vi "Periodic Tasks.vi"(8 "error in (no error)":errorcluster) -> ()   [LabVIEW 2012]
doc: "This VI runs in parallel to other tasks. It can contain as many user-defined periodic loops as you need. These can carry out PID or other sorts of timed response."
uses:
  <vilib>/Rock Robotics/WPI/Joystick/WPI_JoystickButtonState.ctl
  <vilib>/Rock Robotics/WPI/Solenoid/WPI_SolenoidValue.ctl
  <vilib>/Rock Robotics/SystemInterfaces/Utilities/FPGA_UtilitiesLED Source.ctl
  <vilib>/Rock Robotics/SystemInterfaces/Utilities/FPGA_UtilitiesLED State.ctl
  Robot Global Data.vi
  <vilib>/Rock Robotics/WPI/Solenoid/WPI_SolenoidSetEnum.vi
  <vilib>/Rock Robotics/WPI/Joystick/WPI_JoystickGetSetRefNum.vi
  <vilib>/Rock Robotics/WPI/RobotDrive/WPI_RobotDriveGetSetRefNum.vi
  <vilib>/Rock Robotics/WPI/RobotDrive/WPI_RobotDriveArcadeDrive_Standard(NoSaturation).vi
  <vilib>/Rock Robotics/WPI/Compressor/WPI_CompressorGetSetRefNum.vi
panel:
  out "Axes":T1
  out "Buttons":T2
  out "Voltage":dbl
  out "Emergency Stop":bool
  out "rear":bool
  out "front":bool
  out "Right Rear":bool
  out "Left Rear":bool
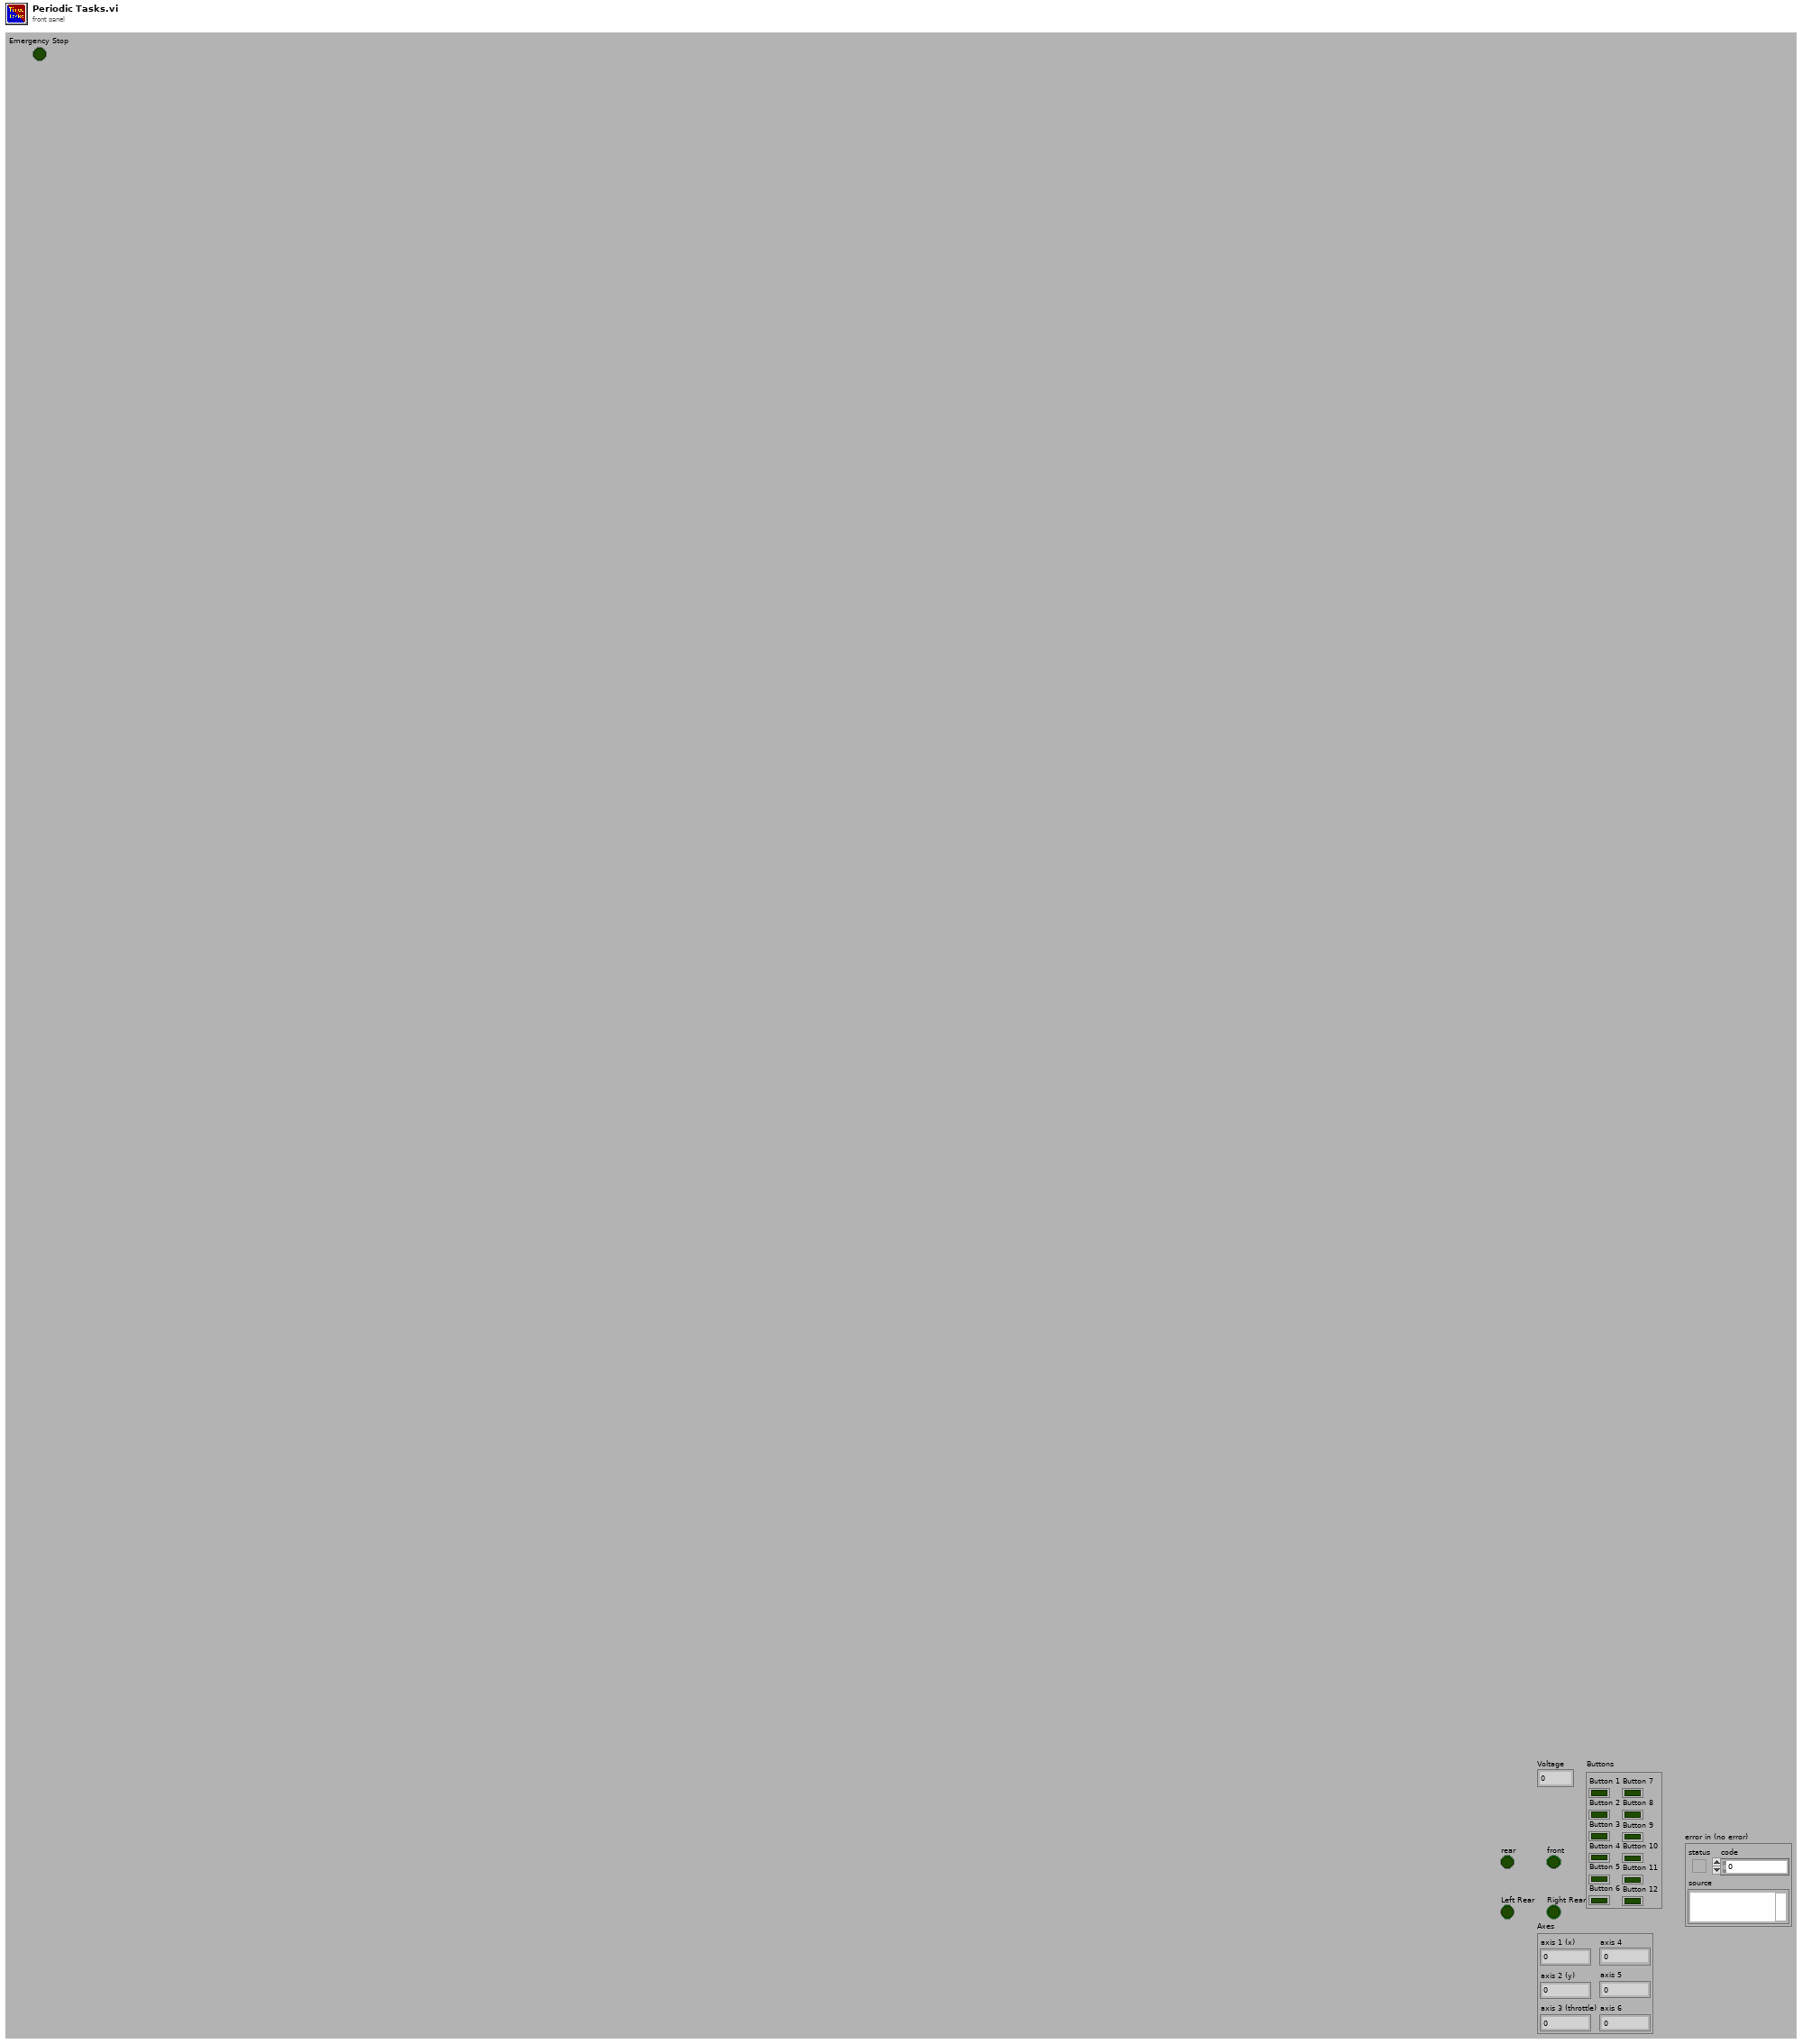
[diagram p1: front panel]
types:
  T1 = cluster{"axis 1 (x)":dbl, "axis 2 (y)":dbl, "axis 3 (throttle)":dbl, "axis 4":dbl, "axis 5":dbl, "axis 6":dbl}
  T2 = typedef "WPI_JoystickButtonState.ctl" = cluster{"Button 1":bool, "Button 2":bool, "Button 3":bool, "Button 4":bool, "Button 5":bool, "Button 6":bool, "Button 7":bool, "Button 8":bool, "Button 9":bool, "Button 10":bool, "Button 11":bool, "Button 12":bool}
  T3 = typedef "WPI_SolenoidValue.ctl" = enum16{"Off", "On", "Forward", "Reverse"}
  T4 = typedef "WPI_MotorControlDeviceRef.ctl" = cluster{"DeviceStatus":errorcluster, "Type":enum16{"PWM", "CAN"}, "PWM":cluster{"Digital Module":T5, "PWM Channel":T6, "DeadBand":T7}, "CAN":cluster{"Device Number":u8, "Control Mode":T8, "Semaphore":T9, "Max Vout":dbl}, "Invert":bool, "TransformRef":T10, "InvTransformRef":T10}
  T5 = typedef "FPGA_TypedefDigitalModule.ctl" = enum16{"Digital Module 1", "Digital Module 2"}
  T6 = typedef "FPGA_DIOPWMChannel.ctl" = enum8{"PWM 1", "PWM 2", "PWM 3", "PWM 4", "PWM 5", "PWM 6", "PWM 7", "PWM 8", "PWM 9", "PWM 10", "Invalid"}
  T7 = typedef "WPI_PWMDeadband.ctl" = cluster{"Name":string, "maxPositivePwm":i32, "minPositivePwm":i32, "centerPwm":i32, "maxNegativePwm":i32, "minNegativePwm":i32, "angularRange":u16}
  T8 = typedef "WPI_CANJaguar_ControlMode.ctl" = enum8{"Percent VBus", "Current", "Speed", "Position", "Voltage"}
  T9 = typedef "Semaphore RefNum" = refnum<k1>
  T10 = typedef "WPI_PWMTransform_ConPane.ctl" = refnum<vi>
  T11 = typedef "WPI_CompressorDevRef.ctl" = cluster{"DevStatus":errorcluster, "DigitalInputDevRef":T12, "RelayDevRef":T14}
  T12 = typedef "WPI_DigitalInputDevRef.ctl" = cluster{"DevStatus":errorcluster, "DIO Channel":T13, "Digital Module":T5}
  T13 = typedef "FPGA_DIOChannel.ctl" = enum8{"DIO 1", "DIO 2", "DIO 3", "DIO 4", "DIO 5", "DIO 6", "DIO 7", "DIO 8", "DIO 9", "DIO 10", "DIO 11", "DIO 12", "DIO 13", "DIO 14", "Invalid"}
  T14 = typedef "WPI_RelayDevRef.ctl" = cluster{"DevStatus":errorcluster, "Relay Channel":T15, "Digital Module":T5, "Relay Direction":T16}
  T15 = typedef "FPGA_DIORelayChannel.ctl" = enum8{"Relay 1", "Relay 2", "Relay 3", "Relay 4", "Relay 5", "Relay 6", "Relay 7", "Relay 8", "Invalid"}
  T16 = typedef "WPI_RelayDirection.ctl" = enum16{"Both directions", "Forward only", "Reverse only"}
  T17 = typedef "WPI_SolenoidDevRef.ctl" = cluster{"DevStatus":errorcluster, "Solenoid Module":T18, "Forward Solenoid Channel":T19, "Reverse Solenoid Channel":T19}
  T18 = typedef "FPGA_TypedefSolenoidModule.ctl" = enum16{"Solenoid Module 1", "Solenoid Module 2"}
  T19 = typedef "WPI_SolenoidChannel.ctl" = enum8{"Solenoid 1", "Solenoid 2", "Solenoid 3", "Solenoid 4", "Solenoid 5", "Solenoid 6", "Solenoid 7", "Solenoid 8", "Invalid"}
  T20 = typedef "WPI_JoystickDevRef.ctl" = cluster{"Device":T21}
  T21 = typedef "WPI_JoystickDeviceEnum.ctl" = enum16{"USB 1", "USB 2", "USB 3", "USB 4", "Kinect 1", "Kinect 2"}
  T22 = typedef "WPI_AnalogChannelDevRef.ctl" = cluster{"DevStatus":errorcluster, "Analog Module":T23, "Analog Channel":T24}
  T23 = typedef "FPGA_TypedefAnalogModule.ctl" = enum16{"Analog Module 1", "Analog Module 2"}
  T24 = typedef "FPGA_AIChannel.ctl" = enum8{"AI 1", "AI 2", "AI 3", "AI 4", "AI 5", "AI 6", "AI 7", "AI 8", "Invalid"}
  T25 = typedef "WPI_RobotDriveDevRef.ctl" = cluster{"DevStatus":errorcluster, "Motors[]":T4[], "Square Inputs":bool, "Max Output":dbl, "Isochronous":bool}
  T26 = typedef "FPGA_UtilitiesLED State.ctl" = enum16{"Off", "On", "Toggle"}
  T27 = typedef "FPGA_UtilitiesLED Source.ctl" = enum16{"User LED", "FPGA LED"}
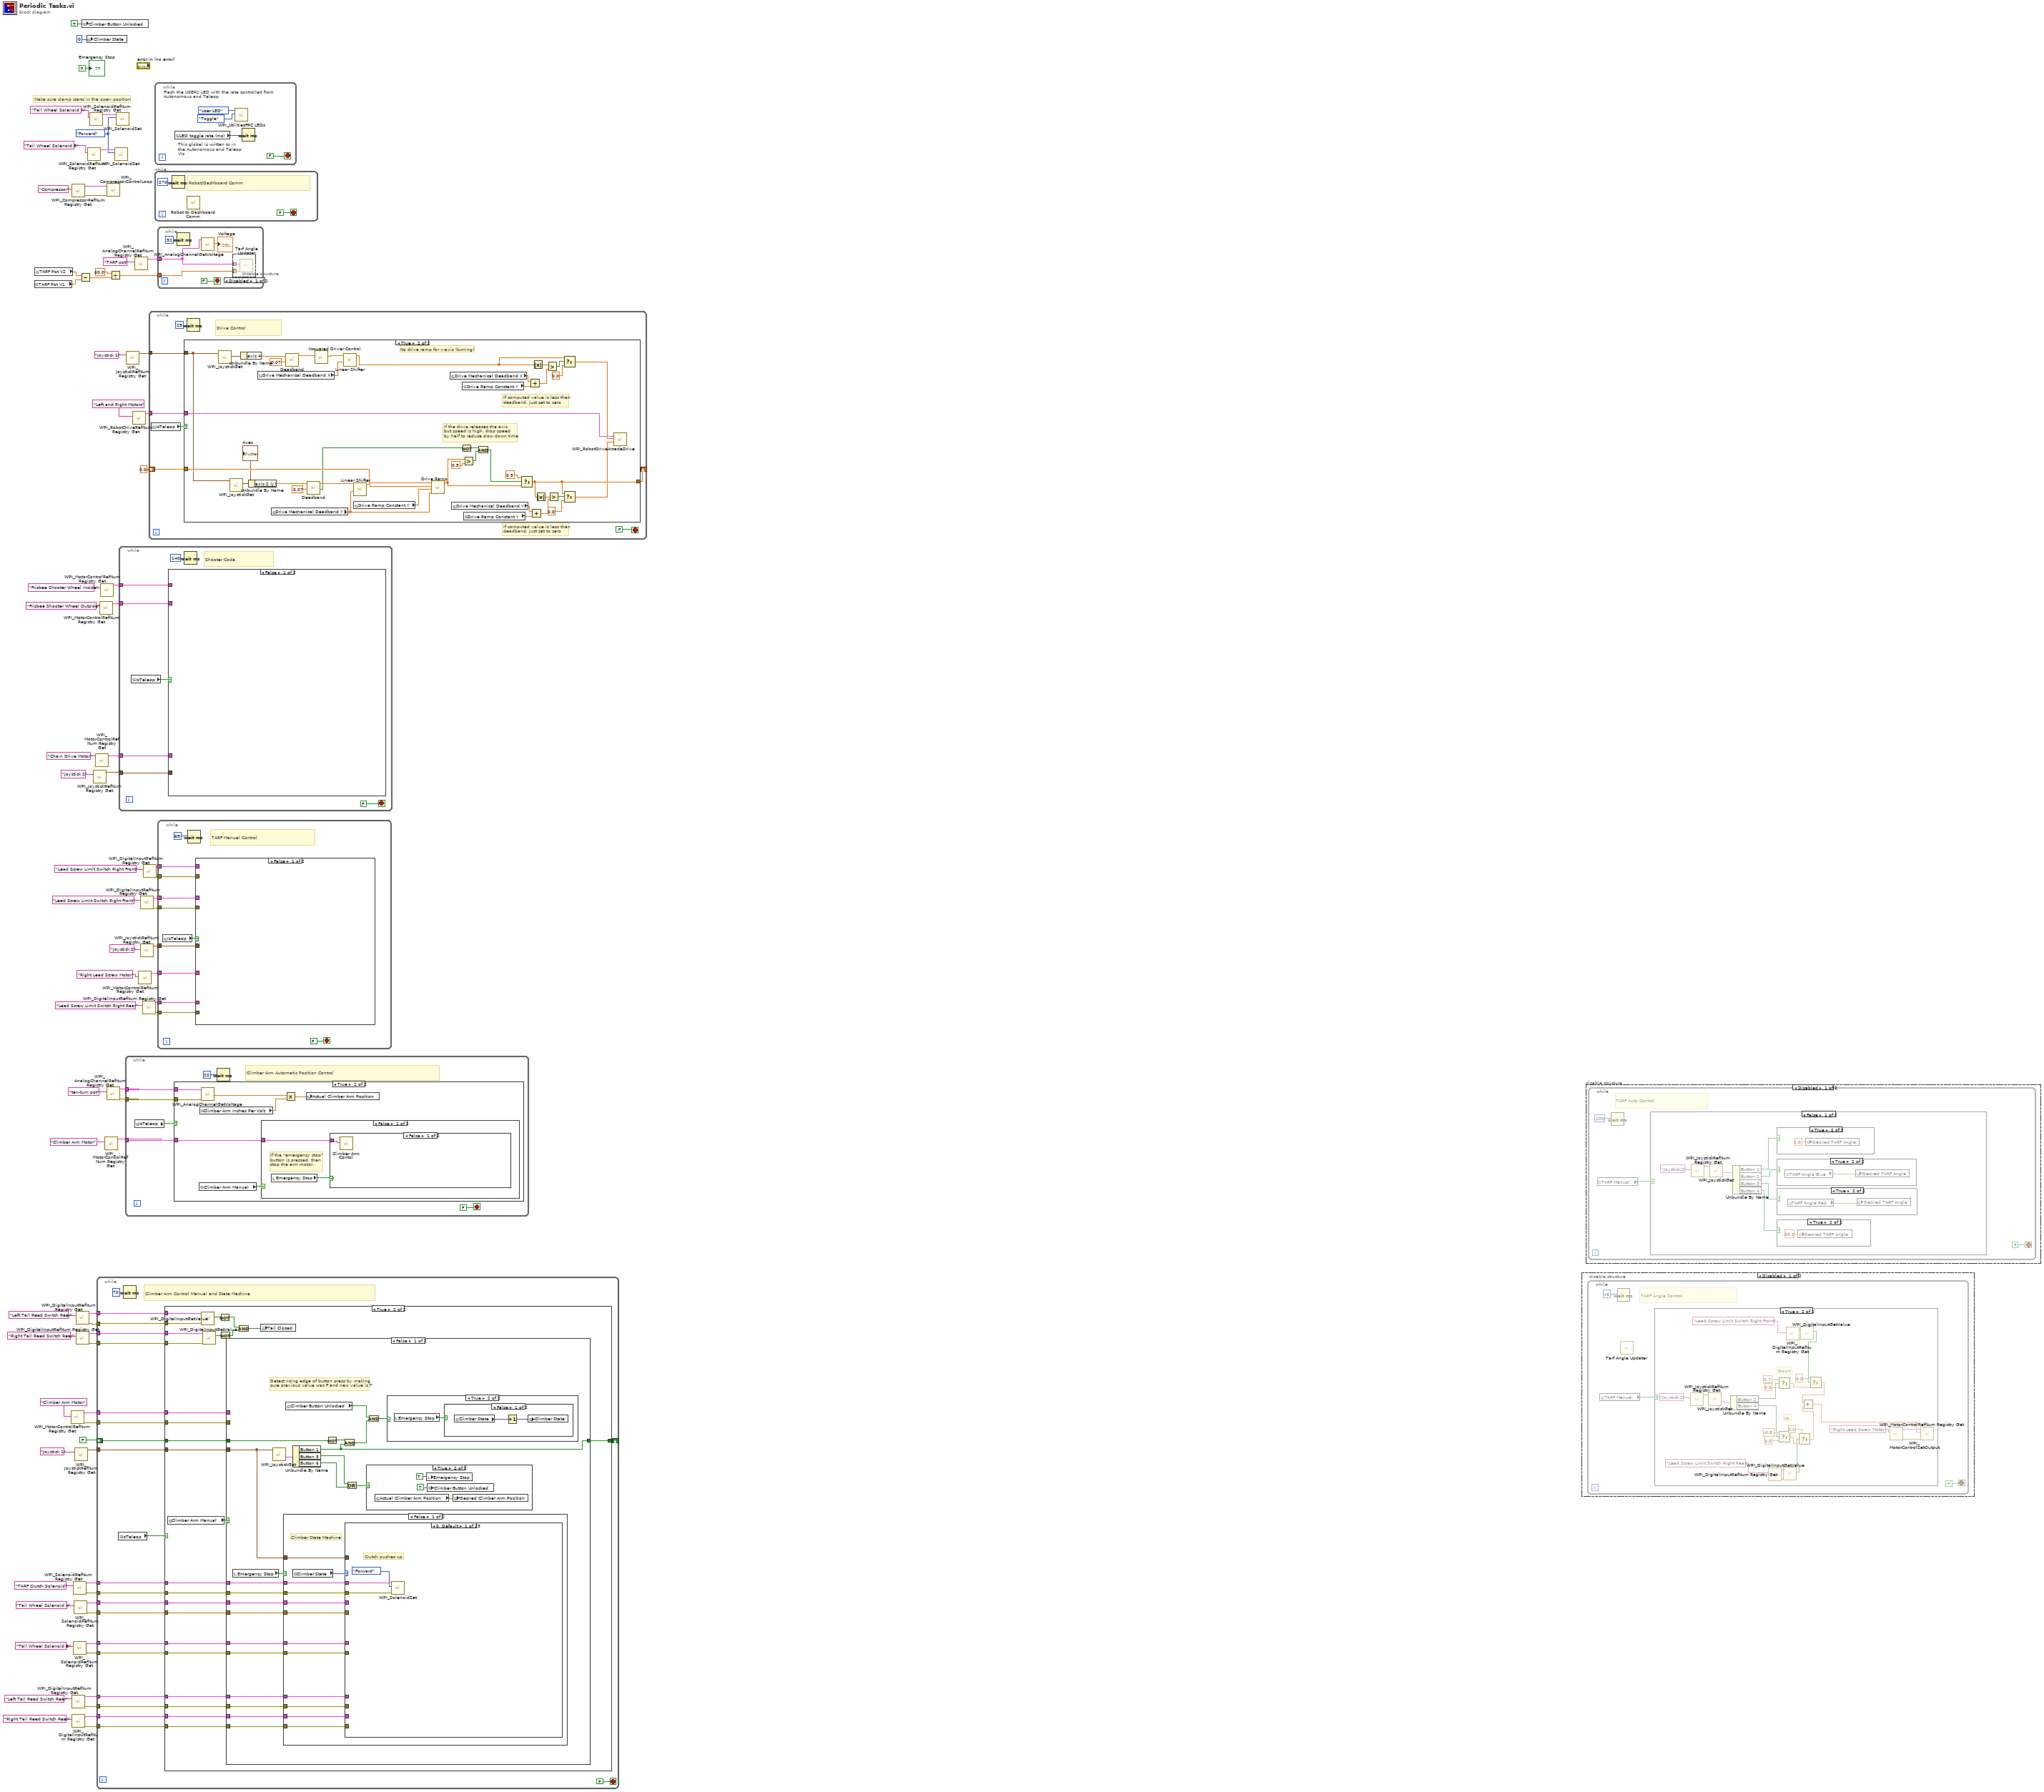
[diagram p0: block diagram]
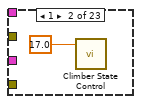
[diagram p4: hidden frame]
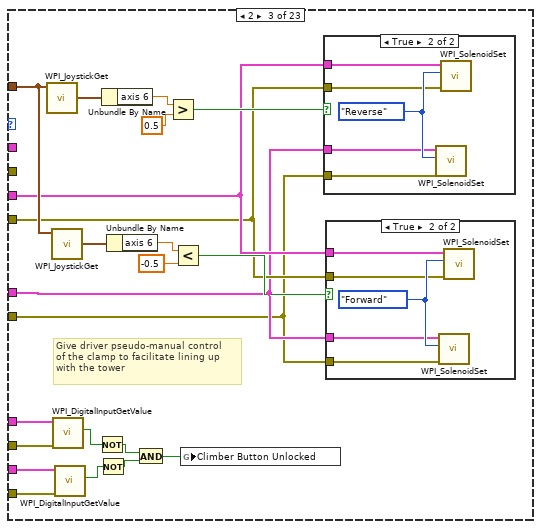
[diagram p5: hidden frame]
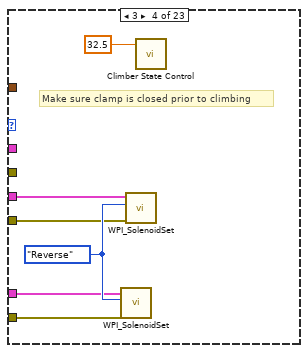
[diagram p8: hidden frame]
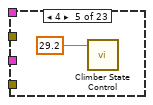
[diagram p9: hidden frame]
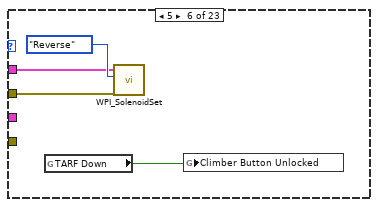
[diagram p10: hidden frame]
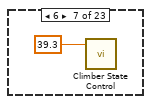
[diagram p11: hidden frame]
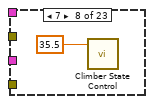
[diagram p12: hidden frame]
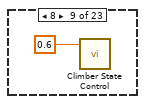
[diagram p13: hidden frame]
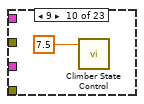
[diagram p14: hidden frame]
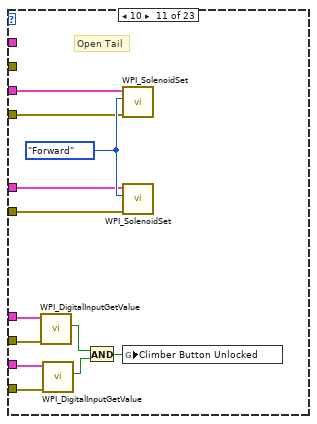
[diagram p15: hidden frame]
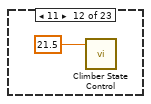
[diagram p16: hidden frame]
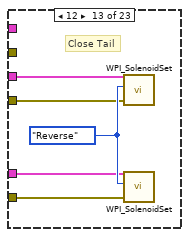
[diagram p17: hidden frame]
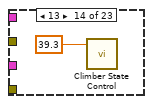
[diagram p18: hidden frame]
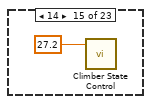
[diagram p19: hidden frame]
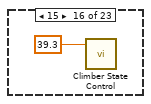
[diagram p20: hidden frame]
diagram:
  w67 = WPI_SolenoidValue."Forward" ("Value")
  # "Make sure clamp starts in the open position"
  n1 = global read "Robot Global Data.vi" "TARF Pot V1"() -> (w4:dbl)
  n2 = global read "Robot Global Data.vi" "TARF Pot V2"() -> (w5:dbl)
  n3 = call <vilib>:"WPI_MotorControlRefNum Registry Get.vi"("refnum name"="Climber Arm Motor") -> ("error out"=w8:errorcluster, "MotorControlDevRef"=w9:T4)  [unwired: 9 in]
  n4 = call <vilib>:"WPI_CompressorRefNum Registry Get.vi"("refnum name"="Compressor") -> ("error out"=w75:errorcluster, "CompressorDevRef"=w76:T11)  [unwired: 9 in]
  n5 = call <vilib>:"WPI_DigitalInputRefNum Registry Get.vi"("refnum name"="Left Tail Reed Switch Rear") -> ("error out"=w13:errorcluster, "DigitalInputDevRef"=w14:T12)  [unwired: 9 in]
  n6 = call <vilib>:"WPI_DigitalInputRefNum Registry Get.vi"("refnum name"="Right Tail Reed Switch Rear") -> ("error out"=w11:errorcluster, "DigitalInputDevRef"=w12:T12)  [unwired: 9 in]
  n7 = call <vilib>:"WPI_SolenoidRefNum Registry Get.vi"("refnum name"="TARF Crutch Solenoid") -> ("error out"=w17:errorcluster, "SolenoidDevRef"=w18:T17)  [unwired: 9 in]
  n8 = call <vilib>:"WPI_SolenoidRefNum Registry Get.vi"("refnum name"="Tail Wheel Solenoid B") -> ("error out"=w20:errorcluster, "SolenoidDevRef"=w21:T17)  [unwired: 9 in]
  n9 = call <vilib>:"WPI_SolenoidRefNum Registry Get.vi"("refnum name"="Tail Wheel Solenoid A") -> ("error out"=w22:errorcluster, "SolenoidDevRef"=w23:T17)  [unwired: 9 in]
  n10 = call <vilib>:"WPI_JoystickRefNum Registry Get.vi"("refnum name"="Joystick 1") -> ("JoystickDevRef"=w26:T20)  [unwired: 9 in, 1 out]
  n11 = call <vilib>:"WPI_DigitalInputRefNum Registry Get.vi"("refnum name"="Left Tail Reed Switch Rear") -> ("error out"=w30:errorcluster, "DigitalInputDevRef"=w31:T12)  [unwired: 9 in]
  n12 = call <vilib>:"WPI_DigitalInputRefNum Registry Get.vi"("refnum name"="Right Tail Reed Switch Rear") -> ("error out"=w28:errorcluster, "DigitalInputDevRef"=w29:T12)  [unwired: 9 in]
  n13 = Subtract(x=w5, y=w4) -> (x-y=w3:dbl)
  n14 = global write "Robot Global Data.vi" "Climber Button Unlocked"(TRUE ("Climber Button Unlocked")) -> ()
  n15 = global write "Robot Global Data.vi" "Climber State"(u8 0 ("Climber State")) -> ()
  n16 = call <vilib>:"WPI_SolenoidRefNum Registry Get.vi"("refnum name"="Tail Wheel Solenoid B") -> ("SolenoidDevRef"=w68:T17)  [unwired: 9 in, 1 out]
  n17 = call <vilib>:"WPI_SolenoidRefNum Registry Get.vi"("refnum name"="Tail Wheel Solenoid A") -> ("SolenoidDevRef"=w70:T17)  [unwired: 9 in, 1 out]
  n18 = call <vilib>:"WPI_JoystickRefNum Registry Get.vi"("refnum name"="Joystick 2") -> ("JoystickDevRef"=w59:T20)  [unwired: 9 in, 1 out]
  n19 = call <vilib>:"WPI_MotorControlRefNum Registry Get.vi"("refnum name"="Chain Drive Motor") -> ("MotorControlDevRef"=w57:T4)  [unwired: 9 in, 1 out]
  n20 = while {
    shift-right: [w96] -> _
    shift-left: FALSE ("Button 1") -> [w95]
    tunnel: w31 -> [w94]
    tunnel: w30 -> [w93]
    tunnel: w29 -> [w92]
    tunnel: w28 -> [w91]
    tunnel: w26 -> [w90]
    tunnel: w23 -> [w89]
    tunnel: w22 -> [w88]
    tunnel: w21 -> [w87]
    tunnel: w20 -> [w86]
    tunnel: w18 -> [w85]
    tunnel: w17 -> [w84]
    tunnel: w14 -> [w83]
    tunnel: w13 -> [w82]
    tunnel: w12 -> [w81]
    tunnel: w11 -> [w80]
    tunnel: w9 -> [w79]
    tunnel: w8 -> [w78]
    stop <- FALSE stop-if-true
    # "Climber Arm Control Manual and State Machine"
    n21 = global read "Robot Global Data.vi" "IsTeleop"() -> (w77:bool)
    n22 = Wait (ms)(milliseconds to wait=u32 70) -> ()  [unwired: 1 out]
    n23 = case shown="True" w77 {
      tunnel: [w99 w123] -> w96
      tunnel: w95 -> [w99 w122]
      tunnel: w94 -> [_ w116]
      tunnel: w93 -> [_ w115]
      tunnel: w92 -> [_ w114]
      tunnel: w91 -> [_ w113]
      tunnel: w90 -> [_ w112]
      tunnel: w89 -> [_ w111]
      tunnel: w88 -> [_ w110]
      tunnel: w87 -> [_ w109]
      tunnel: w86 -> [_ w108]
      tunnel: w85 -> [_ w107]
      tunnel: w84 -> [_ w106]
      tunnel: w83 -> [_ w105]
      tunnel: w82 -> [_ w104]
      tunnel: w81 -> [_ w103]
      tunnel: w80 -> [_ w102]
      tunnel: w79 -> [_ w101]
      tunnel: w78 -> [_ w100]
      frame False {
      }
      frame True {
        n24 = global read "Robot Global Data.vi" "Climber Arm Manual"() -> (w124:bool)
        n25 = call <vilib>:"WPI_DigitalInputGetValue.vi"("error in (no error)"=w115, "DigitalInputDevRef"=w116) -> ("Value"=w120:bool)  [unwired: 7 in, 2 out]
        n26 = call <vilib>:"WPI_DigitalInputGetValue.vi"("error in (no error)"=w113, "DigitalInputDevRef"=w114) -> ("Value"=w119:bool)  [unwired: 7 in, 2 out]
        n27 = Not(x=w120) -> (.not. x?=w117:bool)
        n28 = Not(x=w119) -> (.not. x?=w118:bool)
        n29 = case shown="False" w124 {
          tunnel: [w141 w284] -> w123
          tunnel: w122 -> [w140 w284]
          tunnel: w112 -> [w125 w268]
          tunnel: w111 -> [w135 w264]
          tunnel: w110 -> [w134 w263]
          tunnel: w109 -> [w133 w262]
          tunnel: w108 -> [w132 w261]
          tunnel: w107 -> [w131 _]
          tunnel: w106 -> [w130 _]
          tunnel: w105 -> [w129 _]
          tunnel: w104 -> [w128 _]
          tunnel: w103 -> [w127 _]
          tunnel: w102 -> [w126 _]
          tunnel: w101 -> [_ w267]
          tunnel: w100 -> [_ w266]
          frame False {
            # "Detect rising edge of button press by making\nsure previous value was F and new value is T"
            n30 = local read "Emergency Stop"() -> (w143:bool)
            n31 = call <vilib>:"WPI_JoystickGet.vi"("JoystickDevRef"=w125) -> ("Buttons"=w146:T2)  [unwired: 4 in, 2 out]
            n32 = case shown="False" w143 {
              tunnel: w135 -> [w157 _]
              tunnel: w134 -> [w156 _]
              tunnel: w133 -> [w155 _]
              tunnel: w132 -> [w154 _]
              tunnel: w131 -> [w153 _]
              tunnel: w130 -> [w152 _]
              tunnel: w125 -> [w151 _]
              tunnel: w129 -> [w150 _]
              tunnel: w128 -> [w149 _]
              tunnel: w127 -> [w148 _]
              tunnel: w126 -> [w147 _]
              frame False {
                # "Climber State Machine"
                n33 = global read "Robot Global Data.vi" "Climber State"() -> (w158:u8)
                n34 = case shown="0, Default" w158 {
                  tunnel: w157 -> [_ _ w170 w198 _ _ _ _ _ _ w217 _ w226 _ _ _ _ _ w240 _ w249 _ _]
                  tunnel: w156 -> [_ _ w169 w197 _ _ _ _ _ _ w216 _ w225 _ _ _ _ _ w239 _ w248 _ _]
                  tunnel: w155 -> [_ _ w168 w196 _ _ _ _ _ _ w211 _ w224 _ _ _ _ _ w238 _ w247 _ _]
                  tunnel: w154 -> [_ _ w167 w195 _ _ _ _ _ _ w210 _ w223 _ _ _ _ _ w237 _ w246 _ _]
                  tunnel: w153 -> [w160 _ _ _ _ w203 _ _ _ _ _ _ _ _ _ _ _ _ _ _ _ _ _]
                  tunnel: w152 -> [w159 _ _ _ _ w202 _ _ _ _ _ _ _ _ _ _ _ _ _ _ _ _ _]
                  tunnel: w151 -> [_ _ w171 _ _ _ _ _ _ _ _ _ _ _ _ _ _ _ _ _ _ _ _]
                  tunnel: w150 -> [_ _ w166 _ _ _ _ _ _ _ w215 _ _ _ _ _ _ _ w236 _ _ _ _]
                  tunnel: w149 -> [_ _ w165 _ _ _ _ _ _ _ w214 _ _ _ _ _ _ _ w235 _ _ _ _]
                  tunnel: w148 -> [_ _ w164 _ _ _ _ _ _ _ w213 _ _ _ _ _ _ _ w234 _ _ _ _]
                  tunnel: w147 -> [_ _ w163 _ _ _ _ _ _ _ w212 _ _ _ _ _ _ _ w233 _ _ _ _]
                  frame 0, Default {
                    # "Crutch pushes up"
                    n35 = call-poly <vilib>:"WPI_SolenoidSet.vi"("error in (no error)"=w159, "Value"=WPI_SolenoidValue."Forward", "SolenoidDevRef"=w160) -> ()  [unwired: 7 in, 2 out]
                  }
                  frame 1 {
                    n36 = call "Climber State Control.vi"("Desired Position"=17.0 ("Desired Angle")) -> ()  [unwired: 11 in]
                  }
                  frame 2 {
                    # "Give driver pseudo-manual control\nof the clamp to facilitate lining up\nwith the tower"
                    n37 = call <vilib>:"WPI_JoystickGet.vi"("JoystickDevRef"=w171) -> ("Axes"=w184:T1)  [unwired: 4 in, 2 out]
                    n38 = call <vilib>:"WPI_JoystickGet.vi"("JoystickDevRef"=w171) -> ("Axes"=w180:T1)  [unwired: 4 in, 2 out]
                    n39 = call <vilib>:"WPI_DigitalInputGetValue.vi"("error in (no error)"=w165, "DigitalInputDevRef"=w166) -> ("Value"=w173:bool)  [unwired: 7 in, 2 out]
                    n40 = call <vilib>:"WPI_DigitalInputGetValue.vi"("error in (no error)"=w163, "DigitalInputDevRef"=w164) -> ("Value"=w174:bool)  [unwired: 7 in, 2 out]
                    n41 = Not(x=w173) -> (.not. x?=w172:bool)
                    n42 = Not(x=w174) -> (.not. x?=w175:bool)
                    n43 = Unbundle By Name(w184) -> ("axis 6"=w183:dbl)
                    n44 = Unbundle By Name(w180) -> ("axis 6"=w179:dbl)
                    n45 = And(x=w172, y=w175) -> (x .and. y?=w176:bool)
                    n46 = Greater?(x=w183, y=0.5) -> (0:w181:bool)
                    n47 = Less?(x=w179, y=-0.5) -> (x < y?=w177:bool)
                    n48 = global write "Robot Global Data.vi" "Climber Button Unlocked"(w176) -> ()
                    n49 = case shown="True" w181 {
                      tunnel: w170 -> [_ w193]
                      tunnel: w169 -> [_ w192]
                      tunnel: w168 -> [_ w191]
                      tunnel: w167 -> [_ w190]
                      frame False {
                      }
                      frame True {
                        w194 = WPI_SolenoidValue."Reverse" ("Value")
                        n50 = call-poly <vilib>:"WPI_SolenoidSet.vi"("error in (no error)"=w190, "Value"=w194, "SolenoidDevRef"=w191) -> ()  [unwired: 7 in, 2 out]
                        n51 = call-poly <vilib>:"WPI_SolenoidSet.vi"("error in (no error)"=w192, "Value"=w194, "SolenoidDevRef"=w193) -> ()  [unwired: 7 in, 2 out]
                      }
                    }
                    n52 = case shown="True" w177 {
                      tunnel: w170 -> [_ w188]
                      tunnel: w169 -> [_ w187]
                      tunnel: w168 -> [_ w186]
                      tunnel: w167 -> [_ w185]
                      frame False {
                      }
                      frame True {
                        w189 = WPI_SolenoidValue."Forward" ("Value")
                        n53 = call-poly <vilib>:"WPI_SolenoidSet.vi"("error in (no error)"=w185, "Value"=w189, "SolenoidDevRef"=w186) -> ()  [unwired: 7 in, 2 out]
                        n54 = call-poly <vilib>:"WPI_SolenoidSet.vi"("error in (no error)"=w187, "Value"=w189, "SolenoidDevRef"=w188) -> ()  [unwired: 7 in, 2 out]
                      }
                    }
                  }
                  frame 3 {
                    w199 = WPI_SolenoidValue."Reverse" ("Value")
                    # "Make sure clamp is closed prior to climbing"
                    n55 = call-poly <vilib>:"WPI_SolenoidSet.vi"("error in (no error)"=w195, "Value"=w199, "SolenoidDevRef"=w196) -> ()  [unwired: 7 in, 2 out]
                    n56 = call-poly <vilib>:"WPI_SolenoidSet.vi"("error in (no error)"=w197, "Value"=w199, "SolenoidDevRef"=w198) -> ()  [unwired: 7 in, 2 out]
                    n57 = call "Climber State Control.vi"("Desired Position"=32.5 ("Desired Angle")) -> ()  [unwired: 11 in]
                  }
                  frame 4 {
                    n58 = call "Climber State Control.vi"("Desired Position"=29.2 ("Desired Angle")) -> ()  [unwired: 11 in]
                  }
                  frame 5 {
                    n59 = global read "Robot Global Data.vi" "TARF Down"() -> (w205:bool)
                    n60 = call-poly <vilib>:"WPI_SolenoidSet.vi"("error in (no error)"=w202, "Value"=WPI_SolenoidValue."Reverse", "SolenoidDevRef"=w203) -> ()  [unwired: 7 in, 2 out]
                    n61 = global write "Robot Global Data.vi" "Climber Button Unlocked"(w205) -> ()
                  }
                  frame 6 {
                    n62 = call "Climber State Control.vi"("Desired Position"=39.3 ("Desired Angle")) -> ()  [unwired: 11 in]
                  }
                  frame 7 {
                    n63 = call "Climber State Control.vi"("Desired Position"=35.5 ("Desired Angle")) -> ()  [unwired: 11 in]
                  }
                  frame 8 {
                    n64 = call "Climber State Control.vi"("Desired Position"=0.6 ("Desired Angle")) -> ()  [unwired: 11 in]
                  }
                  frame 9 {
                    n65 = call "Climber State Control.vi"("Desired Position"=7.5 ("Desired Angle")) -> ()  [unwired: 11 in]
                  }
                  frame 10 {
                    w221 = WPI_SolenoidValue."Forward" ("Value")
                    # "Open Tail"
                    n66 = call <vilib>:"WPI_DigitalInputGetValue.vi"("error in (no error)"=w214, "DigitalInputDevRef"=w215) -> ("Value"=w219:bool)  [unwired: 7 in, 2 out]
                    n67 = call <vilib>:"WPI_DigitalInputGetValue.vi"("error in (no error)"=w212, "DigitalInputDevRef"=w213) -> ("Value"=w220:bool)  [unwired: 7 in, 2 out]
                    n68 = And(x=w219, y=w220) -> (x .and. y?=w218:bool)
                    n69 = call-poly <vilib>:"WPI_SolenoidSet.vi"("error in (no error)"=w216, "Value"=w221, "SolenoidDevRef"=w217) -> ()  [unwired: 7 in, 2 out]
                    n70 = call-poly <vilib>:"WPI_SolenoidSet.vi"("error in (no error)"=w210, "Value"=w221, "SolenoidDevRef"=w211) -> ()  [unwired: 7 in, 2 out]
                    n71 = global write "Robot Global Data.vi" "Climber Button Unlocked"(w218) -> ()
                  }
                  frame 11 {
                    n72 = call "Climber State Control.vi"("Desired Position"=21.5 ("Desired Angle")) -> ()  [unwired: 11 in]
                  }
                  frame 12 {
                    w227 = WPI_SolenoidValue."Reverse" ("Value")
                    # "Close Tail"
                    n73 = call-poly <vilib>:"WPI_SolenoidSet.vi"("error in (no error)"=w225, "Value"=w227, "SolenoidDevRef"=w226) -> ()  [unwired: 7 in, 2 out]
                    n74 = call-poly <vilib>:"WPI_SolenoidSet.vi"("error in (no error)"=w223, "Value"=w227, "SolenoidDevRef"=w224) -> ()  [unwired: 7 in, 2 out]
                  }
                  frame 13 {
                    n75 = call "Climber State Control.vi"("Desired Position"=39.3 ("Desired Angle")) -> ()  [unwired: 11 in]
                  }
                  frame 14 {
                    n76 = call "Climber State Control.vi"("Desired Position"=27.2 ("Desired Angle")) -> ()  [unwired: 11 in]
                  }
                  frame 15 {
                    n77 = call "Climber State Control.vi"("Desired Position"=39.3 ("Desired Angle")) -> ()  [unwired: 11 in]
                  }
                  frame 16 {
                    n78 = call "Climber State Control.vi"("Desired Position"=0.6 ("Desired Angle")) -> ()  [unwired: 11 in]
                  }
                  frame 17 {
                    n79 = call "Climber State Control.vi"("Desired Position"=7.5 ("Desired Angle")) -> ()  [unwired: 11 in]
                  }
                  frame 18 {
                    w244 = WPI_SolenoidValue."Forward" ("Value")
                    # "Open Tail"
                    n80 = call <vilib>:"WPI_DigitalInputGetValue.vi"("error in (no error)"=w235, "DigitalInputDevRef"=w236) -> ("Value"=w242:bool)  [unwired: 7 in, 2 out]
                    n81 = call <vilib>:"WPI_DigitalInputGetValue.vi"("error in (no error)"=w233, "DigitalInputDevRef"=w234) -> ("Value"=w243:bool)  [unwired: 7 in, 2 out]
                    n82 = And(x=w242, y=w243) -> (x .and. y?=w241:bool)
                    n83 = call-poly <vilib>:"WPI_SolenoidSet.vi"("error in (no error)"=w239, "Value"=w244, "SolenoidDevRef"=w240) -> ()  [unwired: 7 in, 2 out]
                    n84 = call-poly <vilib>:"WPI_SolenoidSet.vi"("error in (no error)"=w237, "Value"=w244, "SolenoidDevRef"=w238) -> ()  [unwired: 7 in, 2 out]
                    n85 = global write "Robot Global Data.vi" "Climber Button Unlocked"(w241) -> ()
                  }
                  frame 19 {
                    n86 = call "Climber State Control.vi"("Desired Position"=21.5 ("Desired Angle")) -> ()  [unwired: 11 in]
                  }
                  frame 20 {
                    w250 = WPI_SolenoidValue."Reverse" ("Value")
                    # "Close Tail"
                    n87 = call-poly <vilib>:"WPI_SolenoidSet.vi"("error in (no error)"=w248, "Value"=w250, "SolenoidDevRef"=w249) -> ()  [unwired: 7 in, 2 out]
                    n88 = call-poly <vilib>:"WPI_SolenoidSet.vi"("error in (no error)"=w246, "Value"=w250, "SolenoidDevRef"=w247) -> ()  [unwired: 7 in, 2 out]
                  }
                  frame 21 {
                    n89 = call "Climber State Control.vi"("Desired Position"=39.3 ("Desired Angle")) -> ()  [unwired: 11 in]
                  }
                  frame 22 {
                    n90 = call "Climber State Control.vi"("Desired Position"=34.5 ("Desired Angle")) -> ()  [unwired: 11 in]
                  }
                }
              }
              frame True {
              }
            }
            n91 = global read "Robot Global Data.vi" "Climber Button Unlocked"() -> (w144:bool)
            n92 = Unbundle By Name(w146) -> ("Button 1"=w141:bool, "Button 5"=w137:bool, "Button 6"=w136:bool)
            n93 = Not(x=w140) -> (.not. x?=w142:bool)
            n94 = And(x=w142, y=w141) -> (x .and. y?=w139:bool)
            n95 = Or(x=w137, y=w136) -> (x .or. y?=w138:bool)
            n96 = case shown="True" w138 {
              frame False {
              }
              frame True {
                n97 = global read "Robot Global Data.vi" "Actual Climber Arm Position"() -> (w255:dbl)
                n98 = local write "Emergency Stop"(TRUE ("Emergency Stop")) -> ()
                n99 = global write "Robot Global Data.vi" "Climber Button Unlocked"(TRUE ("Climber Button Unlocked")) -> ()
                n100 = global write "Robot Global Data.vi" "Desired Climber Arm Position"(w255) -> ()
              }
            }
            n101 = And(x=w144, y=w139) -> (x .and. y?=w145:bool)
            n102 = case shown="True" w145 {
              frame False {
              }
              frame True {
                n103 = local read "Emergency Stop"() -> (w256:bool)
                n104 = case shown="False" w256 {
                  frame False {
                    n105 = global read "Robot Global Data.vi" "Climber State"() -> (w258:u8)
                    n106 = Increment(x=w258) -> (x+1=w257:u8)
                    n107 = global write "Robot Global Data.vi" "Climber State"(w257) -> ()
                  }
                  frame True {
                    # "Don't increment state if coming out\nof emergency stop"
                    n108 = local write "Emergency Stop"(FALSE ("Emergency Stop")) -> ()
                  }
                }
              }
            }
          }
          frame True {
            # "Set the desired equal to actual so the climber arm doesn't start\nmoving suddenly when switched back to automatic control"
            # "Reset the climber state. This is intended only\nfor use if the driver accidentally starts the state\nmachine prematurely. NOT to be used once \nclimbing has begun."
            n109 = call <vilib>:"WPI_JoystickGet.vi"("JoystickDevRef"=w268) -> ("Buttons"=w288:T2, "Axes"=w260:T1)  [unwired: 4 in, 1 out]
            n110 = global write "Robot Global Data.vi" "Climber Arm At Position"(TRUE ("Climber Arm At Position")) -> ()
            n111 = Unbundle By Name(w288) -> ("Button 3"=w287:bool, "Button 1"=w286:bool)
            n112 = Unbundle By Name(w260) -> ("axis 6"=w265:dbl)
            n113 = call <vilib>:"WPI_JoystickGet.vi"("JoystickDevRef"=w268) -> ("Buttons"=w283:T2)  [unwired: 4 in, 2 out]
            n114 = Greater?(x=w265, y=0.5) -> (0:w280:bool)
            n115 = Less?(x=w265, y=-0.5) -> (x < y?=w278:bool)
            n116 = And(x=w287, y=w286) -> (x .and. y?=w289:bool)
            n117 = Unbundle By Name(w283) -> ("Button 4"=w282:bool)
            n118 = case shown="True" w289 {
              tunnel: w287 -> [w316 _]
              tunnel: w286 -> [w311 _]
              tunnel: w267 -> [w298 w319]
              tunnel: w266 -> [w297 w318]
              frame False {
                n119 = Select(t=1.0, s=w311, f=0.0) -> (s? t:f=w305:dbl)
                n120 = Select(t=-1.0, s=w316, f=0.0) -> (s? t:f=w306:dbl)
                n121 = global read "Robot Global Data.vi" "Actual Climber Arm Position"() -> (w303:dbl)
                n122 = global read "Robot Global Data.vi" "Actual Climber Arm Position"() -> (w300:dbl)
                n123 = global read "Robot Global Data.vi" "Soft Stop Min"() -> (w304:dbl)
                n124 = global read "Robot Global Data.vi" "Soft Stop Max"() -> (w301:dbl)
                n125 = Less Or Equal?(x=w303, y=w304) -> (x <= y?=w302:bool)
                n126 = Greater Or Equal?(x=w300, y=w301) -> (x >= y?=w299:bool)
                n127 = Select(t=0.0, s=w302, f=w306) -> (s? t:f=w307:dbl)
                n128 = Select(t=0.0, s=w299, f=w305) -> (s? t:f=w308:dbl)
                n129 = Add(x=w307, y=w308) -> (x+y=w317:dbl)
                n130 = call <vilib>:"WPI_MotorControlSetOutput.vi"("error in (no error)"=w297, "Output"=w317, "MotorControlDevRef"=w298) -> ()  [unwired: 6 in, 3 out]
              }
              frame True {
                n131 = call <vilib>:"WPI_MotorControlSetOutput.vi"("error in (no error)"=w318, "Output"=0.0, "MotorControlDevRef"=w319) -> ()  [unwired: 6 in, 3 out]
              }
            }
            n132 = case shown="True" w280 {
              tunnel: w264 -> [_ w324]
              tunnel: w263 -> [_ w323]
              tunnel: w262 -> [_ w322]
              tunnel: w261 -> [_ w321]
              frame False {
              }
              frame True {
                w325 = WPI_SolenoidValue."Reverse" ("Value")
                n133 = call-poly <vilib>:"WPI_SolenoidSet.vi"("error in (no error)"=w321, "Value"=w325, "SolenoidDevRef"=w322) -> ()  [unwired: 7 in, 2 out]
                n134 = call-poly <vilib>:"WPI_SolenoidSet.vi"("error in (no error)"=w323, "Value"=w325, "SolenoidDevRef"=w324) -> ()  [unwired: 7 in, 2 out]
              }
            }
            n135 = case shown="True" w278 {
              tunnel: w264 -> [_ w293]
              tunnel: w263 -> [_ w292]
              tunnel: w262 -> [_ w291]
              tunnel: w261 -> [_ w290]
              frame False {
              }
              frame True {
                w294 = WPI_SolenoidValue."Forward" ("Value")
                n136 = call-poly <vilib>:"WPI_SolenoidSet.vi"("error in (no error)"=w290, "Value"=w294, "SolenoidDevRef"=w291) -> ()  [unwired: 7 in, 2 out]
                n137 = call-poly <vilib>:"WPI_SolenoidSet.vi"("error in (no error)"=w292, "Value"=w294, "SolenoidDevRef"=w293) -> ()  [unwired: 7 in, 2 out]
              }
            }
            n138 = case shown="True" w282 {
              frame False {
              }
              frame True {
                n139 = global write "Robot Global Data.vi" "Climber State"(u8 0 ("Climber State")) -> ()
                n140 = global write "Robot Global Data.vi" "Climber Button Unlocked"(TRUE ("Climber Button Unlocked")) -> ()
              }
            }
            n141 = global read "Robot Global Data.vi" "Actual Climber Arm Position"() -> (w285:dbl)
            n142 = call <vilib>:"WPI_DigitalInputRefNum Registry Get.vi"("refnum name"="Left Tail Reed Switch Rear") -> ("error out"=w275:errorcluster, "DigitalInputDevRef"=w274:T12)  [unwired: 9 in]
            n143 = call <vilib>:"WPI_DigitalInputRefNum Registry Get.vi"("refnum name"="Right Tail Reed Switch Rear") -> ("error out"=w272:errorcluster, "DigitalInputDevRef"=w273:T12)  [unwired: 9 in]
            n144 = global write "Robot Global Data.vi" "Desired Climber Arm Position"(w285) -> ()
            n145 = call <vilib>:"WPI_DigitalInputGetValue.vi"("error in (no error)"=w275, "DigitalInputDevRef"=w274) -> ("Value"=→"Left Rear":bool)  [unwired: 7 in, 2 out]
            n146 = call <vilib>:"WPI_DigitalInputGetValue.vi"("error in (no error)"=w272, "DigitalInputDevRef"=w273) -> ("Value"=→"Right Rear":bool)  [unwired: 7 in, 2 out]
          }
        }
        n147 = And(x=w117, y=w118) -> (x .and. y?=w121:bool)
        n148 = global write "Robot Global Data.vi" "Tail Closed"(w121) -> ()
      }
    }
  }
  n149 = call <vilib>:"WPI_MotorControlRefNum Registry Get.vi"("refnum name"="Frisbee Shooter Wheel Outside") -> ("MotorControlDevRef"=w53:T4)  [unwired: 9 in, 1 out]
  n150 = call <vilib>:"WPI_MotorControlRefNum Registry Get.vi"("refnum name"="Frisbee Shooter Wheel Inside") -> ("MotorControlDevRef"=w54:T4)  [unwired: 9 in, 1 out]
  n151 = call <vilib>:"WPI_MotorControlRefNum Registry Get.vi"("refnum name"="Climber Arm Motor") -> ("MotorControlDevRef"=w35:T4)  [unwired: 9 in, 1 out]
  n152 = call <vilib>:"WPI_AnalogChannelRefNum Registry Get.vi"("refnum name"="ten-turn pot") -> ("error out"=w37:errorcluster, "AIDeviceRef"=w38:T22)  [unwired: 9 in]
  n153 = call <vilib>:"WPI_CompressorControlLoop.vi"("error in (no error)"=w75, "CompressorDevRef"=w76) -> ()  [unwired: 10 in]
  n154 = Divide(x=60.0, y=w3) -> (x/y=w1:dbl)
  n155 = call-poly <vilib>:"WPI_SolenoidSet.vi"("Value"=w67, "SolenoidDevRef"=w68) -> ()  [unwired: 8 in, 2 out]
  n156 = call-poly <vilib>:"WPI_SolenoidSet.vi"("Value"=w67, "SolenoidDevRef"=w70) -> ()  [unwired: 8 in, 2 out]
  n157 = while {
    tunnel: w59 -> [w331]
    tunnel: w57 -> [w330]
    tunnel: w54 -> [w329]
    tunnel: w53 -> [w328]
    stop <- FALSE stop-if-true
    # "Shooter Code"
    n158 = global read "Robot Global Data.vi" "IsTeleop"() -> (w326:bool)
    n159 = case shown="False" w326 {
      tunnel: w331 -> [_ w336]
      tunnel: w330 -> [_ w335]
      tunnel: w329 -> [_ w334]
      tunnel: w328 -> [_ w333]
      frame False {
      }
      frame True {
        # "Regular shooting"
        # "Dump at top of tower"
        n160 = call <vilib>:"WPI_JoystickGet.vi"("JoystickDevRef"=w336) -> ("Buttons"=w357:T2, "Axes"=w352:T1)  [unwired: 4 in, 1 out]
        n161 = Unbundle By Name(w352) -> ("axis 3 (throttle)"=w349:dbl)
        n162 = Unbundle By Name(w357) -> ("Button 5"=w346:bool, "Button 6"=w356:bool)
        n163 = global read "Robot Global Data.vi" "Dump Speed Outside"() -> (w337:dbl)
        n164 = Greater?(x=w349, y=0.1) -> (0:w344:bool)
        n165 = Select(t=-1.0, s=w356, f=0.0) -> (s? t:f=w353:dbl)
        n166 = global read "Robot Global Data.vi" "Dump Speed Inside"() -> (w338:dbl)
        n167 = call <vilib>:"WPI_MotorControlSetOutput.vi"("Output"=w353, "MotorControlDevRef"=w335) -> ()  [unwired: 7 in, 3 out]
        n168 = Select(t=w338, s=w344, f=0.0) -> (s? t:f=w341:dbl)
        n169 = Select(t=w337, s=w344, f=0.0) -> (s? t:f=w343:dbl)
        n170 = Select(t=11.5, s=w346, f=0.0) -> (s? t:f=w339:dbl)
        n171 = Add(x=w341, y=w339) -> (x+y=w340:dbl)
        n172 = Add(x=w343, y=w339) -> (x+y=w342:dbl)
        n173 = call <vilib>:"WPI_MotorControlSetOutput.vi"("Output"=w340, "MotorControlDevRef"=w334) -> ()  [unwired: 7 in, 3 out]
        n174 = call <vilib>:"WPI_MotorControlSetOutput.vi"("Output"=w342, "MotorControlDevRef"=w333) -> ()  [unwired: 7 in, 3 out]
      }
    }
    n175 = Wait (ms)(milliseconds to wait=u32 140) -> ()  [unwired: 1 out]
  }
  n176 = while {
    tunnel: w38 -> [w361]
    tunnel: w37 -> [w360]
    tunnel: w35 -> [w359]
    stop <- FALSE stop-if-true
    # "Climber Arm Automatic Position Control"
    n177 = global read "Robot Global Data.vi" "IsTeleop"() -> (w358:bool)
    n178 = case shown="True" w358 {
      tunnel: w361 -> [_ w366]
      tunnel: w360 -> [_ w365]
      tunnel: w359 -> [_ w364]
      frame False {
      }
      frame True {
        n179 = global read "Robot Global Data.vi" "Climber Arm Manual"() -> (w370:bool)
        n180 = global read "Robot Global Data.vi" "Climber Arm Inches Per Volt"() -> (w368:dbl)
        n181 = call <vilib>:"WPI_AnalogChannelGetVoltage.vi"("error in (no error)"=w365, "AIDeviceRef"=w366) -> ("Voltage"=w369:dbl)  [unwired: 7 in, 2 out]
        n182 = case shown="False" w370 {
          tunnel: w364 -> [w371 _]
          frame False {
            # "If the \"emergency stop\"\nbutton is pressed, then\nstop the arm motor."
            n183 = local read "Emergency Stop"() -> (w372:bool)
            n184 = case shown="False" w372 {
              tunnel: w371 -> [w373 w374]
              frame False {
                n185 = call "Climber Arm Contol.vi"("MotorControlDevRef"=w373) -> ()  [unwired: 11 in]
              }
              frame True {
                # "Set Desired equal to Actual so the motor won't contine to\nmove after the emergency stop button is released"
                n186 = global read "Robot Global Data.vi" "Actual Climber Arm Position"() -> (w375:dbl)
                n187 = call <vilib>:"WPI_MotorControlSetOutput.vi"("Output"=0.0, "MotorControlDevRef"=w374) -> ()  [unwired: 7 in, 3 out]
                n188 = global write "Robot Global Data.vi" "Desired Climber Arm Position"(w375) -> ()
              }
            }
          }
          frame True {
          }
        }
        n189 = Multiply(x=w369, y=w368) -> (x*y=w367:dbl)
        n190 = global write "Robot Global Data.vi" "Actual Climber Arm Position"(w367) -> ()
      }
    }
    n191 = Wait (ms)(milliseconds to wait=u32 20) -> ()  [unwired: 1 out]
  }
  n192 = call <vilib>:"WPI_JoystickRefNum Registry Get.vi"("refnum name"="Joystick 1") -> ("JoystickDevRef"=w63:T20)  [unwired: 1 in, 9 out]
  n193 = call <vilib>:"WPI_RobotDriveRefNum Registry Get.vi"("refnum name"="Left and Right Motors") -> ("RobotDriveDevRef"=w61:T25)  [unwired: 1 in, 9 out]
  n194 = call <vilib>:"WPI_AnalogChannelRefNum Registry Get.vi"("refnum name"="TARF pot") -> ("AIDeviceRef"=w6:T22)  [unwired: 9 in, 1 out]
  n195 = call <vilib>:"WPI_MotorControlRefNum Registry Get.vi"("refnum name"="Right Lead Screw Motor") -> ("MotorControlDevRef"=w40:T4)  [unwired: 9 in, 1 out]
  n196 = call <vilib>:"WPI_DigitalInputRefNum Registry Get.vi"("refnum name"="Lead Screw Limit Switch Right Front") -> ("error out"=w47:errorcluster, "DigitalInputDevRef"=w48:T12)  [unwired: 9 in]
  n197 = call <vilib>:"WPI_JoystickRefNum Registry Get.vi"("refnum name"="Joystick 2") -> ("JoystickDevRef"=w42:T20)  [unwired: 9 in, 1 out]
  n198 = call <vilib>:"WPI_DigitalInputRefNum Registry Get.vi"("refnum name"="Lead Screw Limit Switch Right Rear") -> ("error out"=w44:errorcluster, "DigitalInputDevRef"=w45:T12)  [unwired: 9 in]
  n199 = call <vilib>:"WPI_DigitalInputRefNum Registry Get.vi"("refnum name"="Lead Screw Limit Switch Right Front") -> ("error out"=w50:errorcluster, "DigitalInputDevRef"=w51:T12)  [unwired: 9 in]
  n200 = while {
    shift-right: [w381] -> _
    shift-left: 0.0 ("Drive Mechanical Deadband") -> [w380]
    tunnel: w63 -> [w379]
    tunnel: w61 -> [w378]
    stop <- FALSE stop-if-true
    # "If computed value is less than\ndeadband, just set to zero"
    # "Drive Control"
    n201 = global read "Robot Global Data.vi" "IsTeleop"() -> (w377:bool)
    n202 = case shown="True" w377 {
      tunnel: [w384 w423] -> w381
      tunnel: w380 -> [w384 w422]
      tunnel: w379 -> [_ w386]
      tunnel: w378 -> [_ w385]
      frame False {
      }
      frame True {
        # "If the drive releases the axis,\nbut speed is high, drop speed\nby half to reduce slow down time"
        # "No drive ramp for x-axis (turning)"
        # "If computed value is less than\ndeadband, just set to zero"
        n203 = call <vilib>:"WPI_JoystickGet.vi"("JoystickDevRef"=w386) -> ("Axes"=w414:T1)  [unwired: 1 in, 5 out]
        n204 = call <vilib>:"WPI_JoystickGet.vi"("JoystickDevRef"=w386) -> ("Axes"=w421:T1)  [unwired: 1 in, 5 out]
        "Axes" <- w421
        n205 = Unbundle By Name(w414) -> ("axis 4"=w412:dbl)
        n206 = Unbundle By Name(w421) -> ("axis 2 (y)"=w410:dbl)
        n207 = global read "Robot Global Data.vi" "Drive Mechanical Deadband X"() -> (w408:dbl)
        n208 = global read "Robot Global Data.vi" "Drive Mechanical Deadband Y"() -> (w405:dbl)
        n209 = call "Deadband.vi"("Deadband"=0.07, "Input"=w412) -> ("Output"=w396:dbl)  [unwired: 8 in, 1 out]
        n210 = call "Deadband.vi"("Deadband"=0.07, "Input"=w410) -> ("IsValid"=w389:bool, "Output"=w409:dbl)  [unwired: 8 in]
        n211 = call "Xsquared Driver Control.vi"("joystick input"=w396) -> ("out"=w395:dbl)  [unwired: 10 in]
        n212 = call "Linear Shifter.vi"("Shift"=w408, "Input"=w395) -> ("Output"=w397:dbl)  [unwired: 9 in]
        n213 = call "Linear Shifter.vi"("Shift"=w405, "Input"=w409) -> ("Output"=w407:dbl)  [unwired: 9 in]
        n214 = global read "Robot Global Data.vi" "Drive Ramp Constant Y"() -> (w406:dbl)
        n215 = call "Drive Ramp.vi"("Deadband"=w405, "Ramp Value"=w406, "Control Input"=w407, "Previous Value"=w422) -> ("Next Value"=w391:dbl)  [unwired: 7 in]
        n216 = global read "Robot Global Data.vi" "Drive Mechanical Deadband X"() -> (w402:dbl)
        n217 = global read "Robot Global Data.vi" "Drive Mechanical Deadband Y"() -> (w417:dbl)
        n218 = Not(x=w389) -> (.not. x?=w390:bool)
        n219 = global read "Robot Global Data.vi" "Drive Ramp Constant Y"() -> (w401:dbl)
        n220 = Greater?(x=w391, y=0.5) -> (0:w394:bool)
        n221 = global read "Robot Global Data.vi" "Drive Ramp Constant Y"() -> (w416:dbl)
        n222 = And(x=w390, y=w394) -> (x .and. y?=w392:bool)
        n223 = Select(t=0.5, s=w392, f=w391) -> (s? t:f=w423:dbl)
        n224 = Add(x=w402, y=w401) -> (x+y=w400:dbl)
        n225 = Add(x=w417, y=w416) -> (x+y=w415:dbl)
        n226 = Absolute Value(x=w397) -> (abs(x)=w399:dbl)
        n227 = Absolute Value(x=w423) -> (abs(x)=w420:dbl)
        n228 = Greater?(x=w399, y=w400) -> (0:w398:bool)
        n229 = Greater?(x=w420, y=w415) -> (0:w419:bool)
        n230 = Select(t=w397, s=w398, f=0.0) -> (s? t:f=w387:dbl)
        n231 = Select(t=w423, s=w419, f=0.0) -> (s? t:f=w404:dbl)
        n232 = call-poly <vilib>:"WPI_RobotDriveArcadeDrive.vi"("Y axis value"=w404, "X axis value"=w387, "RobotDriveDevRef"=w385) -> ()  [unwired: 6 in, 3 out]
      }
    }
    n233 = Wait (ms)(milliseconds to wait=u32 25) -> ()  [unwired: 1 out]
  }
  n234 = while {
    stop <- FALSE stop-if-true
    # "This global is written to in the Autonomous and Teleop VIs"
    # "Flash the USER1 LED with the rate controlled from Autonomous and Teleop"
    n235 = global read "Robot Global Data.vi" "LED toggle rate (ms)"() -> (w424:u32)
    n236 = call <vilib>:"WPI_UtilitiesFRC LEDs.vi"("State"=FPGA_UtilitiesLED_State."Toggle", "LED Type"=FPGA_UtilitiesLED_Source."User LED") -> ()  [unwired: 1 in, 9 out]
    n237 = Wait (ms)(milliseconds to wait=w424) -> ()  [unwired: 1 out]
  }
  n238 = while {
    stop <- FALSE stop-if-true
    # "Robot/Dashboard Comm"
    n239 = Wait (ms)(milliseconds to wait=u32 270) -> ()  [unwired: 1 out]
    n240 = call "Robot to Dashboard Comm.vi"() -> ()  [unwired: 12 in]
  }
  n241 = while {
    tunnel: w6 -> [w431]
    tunnel: w1 -> [w433]
    stop <- FALSE stop-if-true
    n242 = Wait (ms)(milliseconds to wait=u32 32) -> ()  [unwired: 1 out]
    n243 = call <vilib>:"WPI_AnalogChannelGetVoltage.vi"("AIDeviceRef"=w431) -> ("Voltage"=→"Voltage":dbl)  [unwired: 8 in, 2 out]
    n244 = disable-structure shown="Disabled" {
      disable-tunnel: w433 -> [w436 _]
      disable-tunnel: w431 -> [w435 _]
      frame Disabled {
        n245 = call "Tarf Angle Updater.vi"("mult"=w436, "AIDeviceRef"=w435) -> ()  [unwired: 10 in]
      }
      frame Enabled {
      }
    }
  }
  n246 = while {
    tunnel: w51 -> [w445]
    tunnel: w50 -> [w444]
    tunnel: w48 -> [w443]
    tunnel: w47 -> [w442]
    tunnel: w45 -> [w441]
    tunnel: w44 -> [w440]
    tunnel: w42 -> [w439]
    tunnel: w40 -> [w438]
    stop <- FALSE stop-if-true
    # "TARF Manual Control"
    n247 = global read "Robot Global Data.vi" "IsTeleop"() -> (w437:bool)
    n248 = Wait (ms)(milliseconds to wait=u32 65) -> ()  [unwired: 1 out]
    n249 = case shown="False" w437 {
      tunnel: w445 -> [_ w455]
      tunnel: w444 -> [_ w454]
      tunnel: w443 -> [_ w453]
      tunnel: w442 -> [_ w452]
      tunnel: w441 -> [_ w451]
      tunnel: w440 -> [_ w450]
      tunnel: w439 -> [_ w449]
      tunnel: w438 -> [_ w448]
      frame False {
      }
      frame True {
        # "Up"
        # "Down"
        n250 = call <vilib>:"WPI_DigitalInputGetValue.vi"("error in (no error)"=w454, "DigitalInputDevRef"=w455) -> ("Value"=w456:bool)  [unwired: 7 in, 2 out]
        n251 = call <vilib>:"WPI_JoystickGet.vi"("JoystickDevRef"=w449) -> ("Buttons"=w472:T2)  [unwired: 4 in, 2 out]
        "Buttons" <- w472
        n252 = call <vilib>:"WPI_DigitalInputGetValue.vi"("error in (no error)"=w450, "DigitalInputDevRef"=w451) -> ("Value"=w461:bool)  [unwired: 7 in, 2 out]
        "rear" <- w461
        n253 = call <vilib>:"WPI_DigitalInputGetValue.vi"("error in (no error)"=w452, "DigitalInputDevRef"=w453) -> ("Value"=w462:bool)  [unwired: 7 in, 2 out]
        "front" <- w462
        n254 = Unbundle By Name(w472) -> ("Button 2"=w470:bool, "Button 4"=w465:bool)
        n255 = global write "Robot Global Data.vi" "TARF Down"(w456) -> ()
        n256 = Select(t=0.5, s=w470, f=0.0) -> (s? t:f=w460:dbl)
        n257 = Select(t=-0.7, s=w465, f=0.0) -> (s? t:f=w458:dbl)
        n258 = Select(t=0.0, s=w462, f=w460) -> (s? t:f=w463:dbl)
        n259 = Select(t=0.0 ("f"), s=w461, f=w458) -> (s? t:f=w464:dbl)
        n260 = Add(x=w463, y=w464) -> (x+y=w471:dbl)
        n261 = call <vilib>:"WPI_MotorControlSetOutput.vi"("Output"=w471, "MotorControlDevRef"=w448) -> ()  [unwired: 7 in, 3 out]
      }
    }
  }
  n262 = disable-structure shown="Disabled" {
    frame Disabled {
      n263 = while {
        stop <- FALSE stop-if-true
        # "TARF Angle Control"
        n264 = global read "Robot Global Data.vi" "TARF Manual"() -> (w473:bool)
        n265 = Wait (ms)(milliseconds to wait=u32 45) -> ()  [unwired: 1 out]
        n266 = call "Tarf Angle Updater.vi"() -> ()  [unwired: 12 in]
        n267 = case shown="True" w473 {
          frame False {
            n268 = disable-structure shown="Disabled" {
              frame Disabled {
                n269 = call "Lead Screw Control.vi"() -> ()  [unwired: 12 in]
              }
              frame Enabled {
              }
            }
          }
          frame True {
            # "Up"
            # "Down"
            n270 = call <vilib>:"WPI_JoystickRefNum Registry Get.vi"("refnum name"="Joystick 2") -> ("JoystickDevRef"=w501:T20)  [unwired: 9 in, 1 out]
            n271 = call <vilib>:"WPI_JoystickGet.vi"("JoystickDevRef"=w501) -> ("Buttons"=w500:T2)  [unwired: 4 in, 2 out]
            n272 = Unbundle By Name(w500) -> ("Button 2"=w495:bool, "Button 4"=w490:bool)
            n273 = call <vilib>:"WPI_DigitalInputRefNum Registry Get.vi"("refnum name"="Lead Screw Limit Switch Right Rear") -> ("error out"=w483:errorcluster, "DigitalInputDevRef"=w482:T12)  [unwired: 9 in]
            n274 = Select(t=0.7, s=w495, f=0.0) -> (s? t:f=w479:dbl)
            n275 = Select(t=-0.8, s=w490, f=0.0) -> (s? t:f=w477:dbl)
            n276 = call <vilib>:"WPI_DigitalInputGetValue.vi"("error in (no error)"=w483, "DigitalInputDevRef"=w482) -> ("Value"=w480:bool)  [unwired: 7 in, 2 out]
            n277 = call <vilib>:"WPI_DigitalInputRefNum Registry Get.vi"("refnum name"="Lead Screw Limit Switch Right Front") -> ("error out"=w487:errorcluster, "DigitalInputDevRef"=w486:T12)  [unwired: 9 in]
            n278 = Select(t=0.0 ("f"), s=w480, f=w477) -> (s? t:f=w489:dbl)
            n279 = call <vilib>:"WPI_DigitalInputGetValue.vi"("error in (no error)"=w487, "DigitalInputDevRef"=w486) -> ("Value"=w485:bool)  [unwired: 7 in, 2 out]
            n280 = Select(t=0.0, s=w485, f=w479) -> (s? t:f=w488:dbl)
            n281 = Add(x=w488, y=w489) -> (x+y=w496:dbl)
            n282 = call <vilib>:"WPI_MotorControlRefNum Registry Get.vi"("refnum name"="Right Lead Screw Motor") -> ("error out"=w497:errorcluster, "MotorControlDevRef"=w498:T4)  [unwired: 9 in]
            n283 = call <vilib>:"WPI_MotorControlSetOutput.vi"("error in (no error)"=w497, "Output"=w496, "MotorControlDevRef"=w498) -> ()  [unwired: 6 in, 3 out]
          }
        }
      }
    }
    frame Enabled {
    }
  }
  n284 = disable-structure shown="Disabled" {
    frame Disabled {
      n285 = while {
        stop <- FALSE stop-if-true
        # "TARF Auto Control"
        n286 = global read "Robot Global Data.vi" "TARF Manual"() -> (w504:bool)
        n287 = Wait (ms)(milliseconds to wait=u32 100) -> ()  [unwired: 1 out]
        n288 = case shown="False" w504 {
          frame False {
            n289 = call <vilib>:"WPI_JoystickRefNum Registry Get.vi"("refnum name"="Joystick 2") -> ("JoystickDevRef"=w511:T20)  [unwired: 9 in, 1 out]
            n290 = call <vilib>:"WPI_JoystickGet.vi"("JoystickDevRef"=w511) -> ("Buttons"=w510:T2)  [unwired: 4 in, 2 out]
            n291 = Unbundle By Name(w510) -> ("Button 1"=w509:bool, "Button 2"=w508:bool, "Button 3"=w507:bool, "Button 4"=w506:bool)
            n292 = case shown="True" w509 {
              frame False {
              }
              frame True {
                n293 = global write "Robot Global Data.vi" "Desired TARF Angle"(1.0 ("Desired TARF Angle")) -> ()
              }
            }
            n294 = case shown="True" w508 {
              frame False {
              }
              frame True {
                n295 = global read "Robot Global Data.vi" "TARF Angle Blue"() -> (w515:dbl)
                n296 = global write "Robot Global Data.vi" "Desired TARF Angle"(w515) -> ()
              }
            }
            n297 = case shown="True" w507 {
              frame False {
              }
              frame True {
                n298 = global read "Robot Global Data.vi" "TARF Angle Red"() -> (w514:dbl)
                n299 = global write "Robot Global Data.vi" "Desired TARF Angle"(w514) -> ()
              }
            }
            n300 = case shown="True" w506 {
              frame False {
              }
              frame True {
                n301 = global write "Robot Global Data.vi" "Desired TARF Angle"(60.0 ("Desired TARF Angle")) -> ()
              }
            }
          }
          frame True {
          }
        }
      }
    }
    frame Enabled {
    }
  }
  "Emergency Stop" <- FALSE ("Emergency Stop")
